vi "ActionVIOnCompile.vi"(8 "error in (no error)":errorcluster, 11 "Device Item Ref in":T1 format="%.0x") -> (0 "error out":errorcluster)   [LabVIEW 2015, in "Modbus Master System Explorer.lvlib"]
uses:
  Modbus Master System Explorer.lvlib
  <vilib>/NI Veristand/Custom Device API/Custom Device Item Ref.ctl
  Shared/Constants.vi
  <vilib>/NI Veristand/Custom Device API/Set Item Property (Variant).vi
  <vilib>/NI VeriStand/Custom Device API/Custom Device API.lvlib
  Shared/Modbus Master Shared.lvlib
  <vilib>/addons/Inline Async API/_Data Access System Explorer/Data Access System Explorer.lvlib
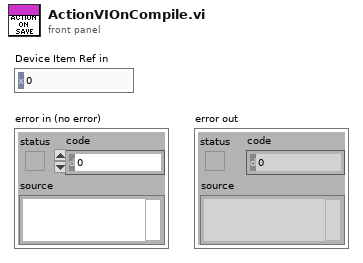
[diagram p1: front panel]
types:
  T1 = typedef "Custom Device API.lvlib/Custom Device Item Ref.ctl" = u64
  T2 = enum16{"Output/Write", "Input/Read", "Input/ReadWrite"}
  T3 = cluster{"Name":string, "Type":enum16{"Output/Write", "Input/Read", "Input/ReadWrite"}, "VS Refs":T1[]}
  T4 = typedef "Modbus Master Shared.lvlib/Device Info.ctl" = cluster{"Interface Data":cluster{"Name":string, "Unit ID":u8, "Refresh Rate":i32, "Interface Type":T5, "TCP Settings":T6, "Serial Settings":T7}, "Modbus Input Groups":T8[], "Modbus Output Groups":T8[], "error in (no error)":errorcluster, "Modbus Input Engine Group Names":string[], "Modbus Output Engine Group Names":string[]}
  T5 = typedef "Modbus Master Shared.lvlib/Interface Type.ctl" = enum16{"TCP Master", "Serial Master", "TCP Slave", "Serial Slave"}
  T6 = typedef "Modbus Master Shared.lvlib/TCP Settings.ctl" = cluster{"Address":string, "Port":u16, "Timeout":i32}
  T7 = typedef "Modbus Master Shared.lvlib/Serial Settings.ctl" = cluster{"VISA resource name":refnum<visa-resource-name>, "baud rate":u32, "parity (even)":u16, "flow control (none)":u16, "serial type":enum16{"RTU", "ASCII"}}
  T8 = typedef "Modbus Master Shared.lvlib/Bulk Data Access.ctl" = cluster{"Modbus Type":T9, "start":u16, "length":u16, "Channel Data":T10[]}
  T9 = typedef "Modbus Master Shared.lvlib/Modbus Type.ctl" = enum16{"Coil", "Discrete Input", "Holding Register", "Input Register"}
  T10 = typedef "Modbus Master Shared.lvlib/Channel.ctl" = cluster{"Name":string, "Modbus Type":T9, "Veristand Type":T11, "Mapping":T12}
  T11 = typedef "Custom Device API.lvlib/Custom Device Channel Type.ctl" = enum16{"Input", "Output"}
  T12 = typedef "Modbus Master Shared.lvlib/Mapping.ctl" = cluster{"DataType":T13, "Starting Address":u16, "Sub-Index (Bool)":u16, "VS Reference":T1}
  T13 = typedef "Modbus Master Shared.lvlib/DataType.ctl" = enum16{"Double", "Single", "I64", "I32", "I16", "I8", "U64", "U32", "U16", "U8", "Boolean"}
  T14 = typedef "Modbus Master Shared.lvlib/Channel Data.ctl" = cluster{"Coils":T10[], "Discrete Inputs":T10[], "Input Registers":T10[], "Holding Registers":T10[]}
  T15 = cluster{"Name":string, "Type":enum16{"Output/Write", "Input/Read", "Input/ReadWrite"}, "VS Refs":T1[]}[]
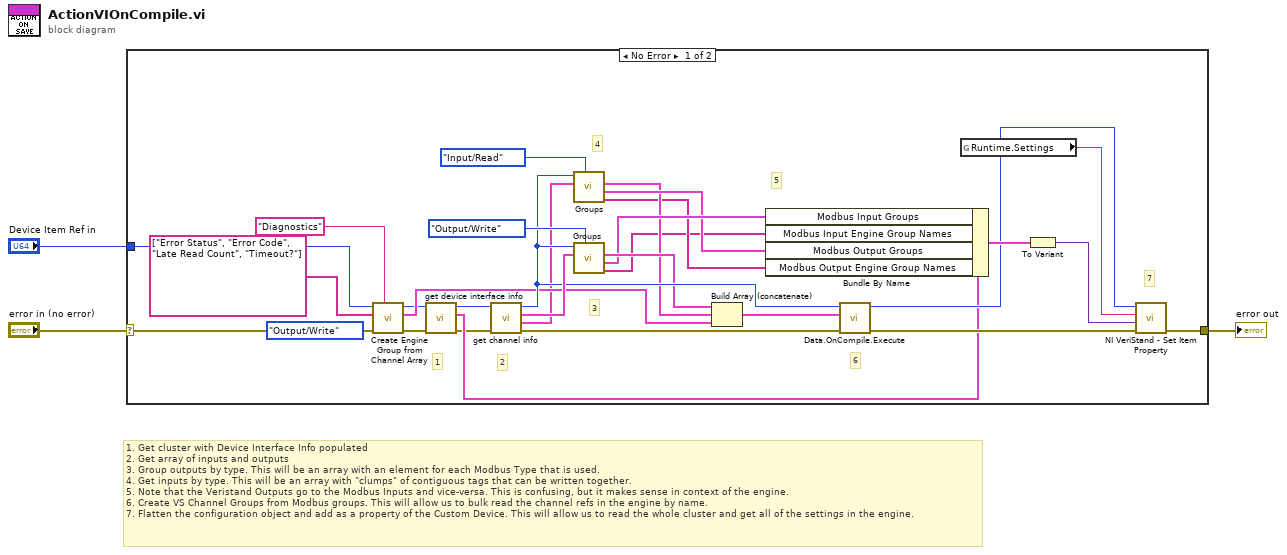
[diagram p0: block diagram]
diagram:
  # "1. Get cluster with Device Interface Info populated\n2. Get array of inputs and outputs\n3. Group outputs by type. This will be an array with an element for each Modbus Type that is used.\n4. Get inputs by type. This will be an array with \"clumps\" of contiguous tags that can be written together.\n5. Note that the Veristand Outputs go to the Modbus Inputs and vice-versa. This is confusing, but it makes sense in context of the engine.\n6. Create VS Channel Groups from Modbus groups. This will allow us to bulk read the channel refs in the engine by name.\n7. Flatten the configuration object and add as a property of the Custom Device. This will allow us to read the whole cluster and get all of the settings in the engine."
  n1 = case shown="No Error" "error in (no error)" {
    selector: "error in (no error)" -> [w14 w34]
    tunnel: [w29 w34] -> w1
    tunnel: "Device Item Ref in" -> [w15 _]
    frame No Error {
      # "5"
      # "7"
      # "6"
      # "4"
      # "3"
      # "2"
      # "1"
      n2 = call "Create Engine Group from Channel Array.vi"("Group Name"="Diagnostics", "error in (no error)"=w14, "Type"=T2."Output/Write", "Item Names"=string[] ["Error Status", "Error Code", "Late Read Count", "Timeout?"], "Device Item Ref in"=w15) -> ("error out"=w9:errorcluster, "output cluster"=w13:T3, "Device Item Ref out"=w10:T1)  [unwired: 4 in]
      n3 = call "get device interface info.vi"("error in (no error)"=w9, "Device Item Ref in in"=w10) -> ("error out"=w21:errorcluster, "Device Info out"=w23:T4, "Device Item Ref out"=w22:T1)  [unwired: 7 in]
      n4 = call "get channel info.vi"("error in (no error)"=w21, "Item Ref in"=w22) -> ("error out"=w27:errorcluster, "Outputs"=w6:T14, "Inputs"=w20:T14, "Item Ref out"=w19:T1)  [unwired: 6 in]
      n5 = call "Groups.vi"("Type"=T2."Input/Read", "Channel Group"=w6, "Item Ref in"=w19) -> ("Engine Group Names"=w5:string[], "Config Groups"=w16:T8[], "Engine Groups"=w7:T15)  [unwired: 5 in, 1 out]
      n6 = call "Groups.vi"("Type"=T2."Output/Write", "Channel Group"=w20, "Item Ref in"=w19) -> ("Engine Group Names"=w4:string[], "Config Groups"=w17:T8[], "Engine Groups"=w18:T15)  [unwired: 5 in, 1 out]
      n7 = Build Array (concatenate)(w18, w7, w13) -> (w24:T15)
      n8 = Bundle By Name(cluster=w23, "Modbus Input Groups"=w17, "Modbus Input Engine Group Names"=w4, "Modbus Output Groups"=w16, "Modbus Output Engine Group Names"=w5) -> (w32:T4)
      n9 = call <vilib>:"Data.OnCompile.Execute.vi"("error in"=w27, "VS Ref Groups"=w24, "Custom Device Ref"=w19) -> ("error out"=w28:errorcluster, "Custom Device Ref"=w30:T1)  [unwired: 7 in]
      n10 = global read "Constants.vi" "Runtime.Settings"() -> (w33:string)
      n11 = To Variant(anything=w32) -> (Variant=w31:variant)
      n12 = call-poly <vilib>:"NI VeriStand - Set Item Property.vi"("error in (no error)"=w28, "Value"=w31, "Property Name"=w33, "Item Ref in"=w30) -> ("error out"=w29:errorcluster)  [unwired: 5 in, 2 out]
    }
    frame Error {
    }
  }
  "error out" <- w1
